vi "9205 Read 2.vi"(8 "error in":errorcluster, 11 "Module Config Selector":i16) -> (0 "error out":errorcluster, 3 "Data Array":sgl[](array[numeric]))   [LabVIEW 2015]
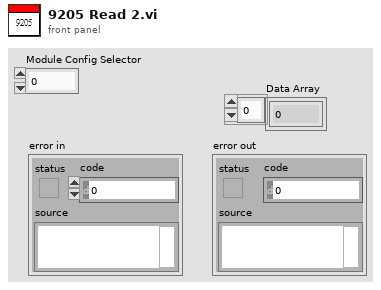
[diagram p1: front panel]
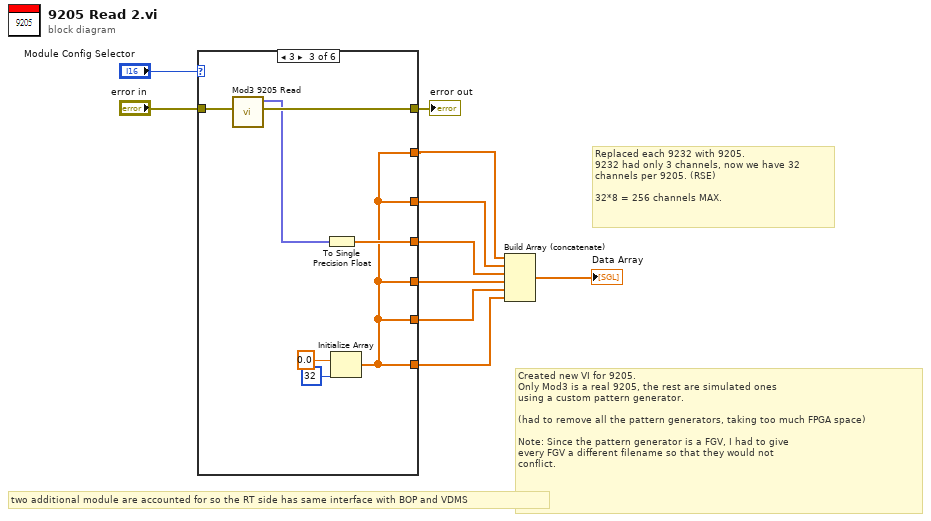
[diagram p0: block diagram]
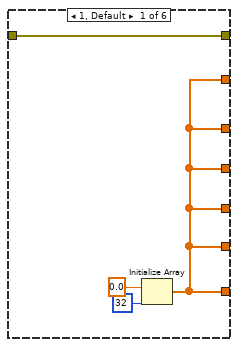
[diagram p2: hidden frame]
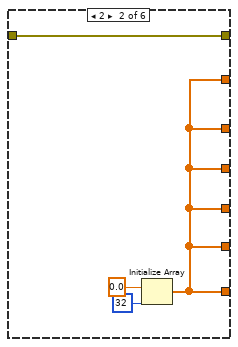
[diagram p3: hidden frame]
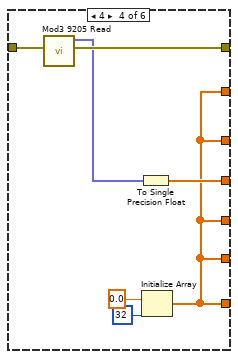
[diagram p4: hidden frame]
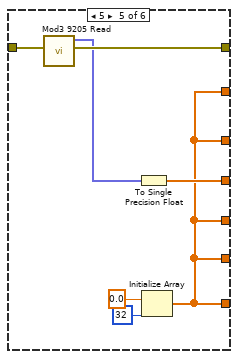
[diagram p5: hidden frame]
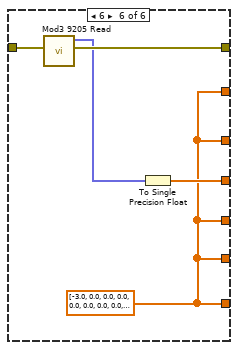
[diagram p6: hidden frame]
diagram:
  # "Replaced each 9232 with 9205.\n9232 had only 3 channels, now we have 32\nchannels per 9205. (RSE)\n\n32*8 = 256 channels MAX."
  # "Created new VI for 9205.\nOnly Mod3 is a real 9205, the rest are simulated ones\nusing a custom pattern generator.\n\n(had to remove all the pattern generators, taking too much FPGA space)\n\nNote: Since the pattern generator is a FGV, I had to give\nevery FGV a different filename so that they would not\nconflict."
  # "two additional module are accounted for so the RT side has same interface with BOP and VDMS"
  n1 = case shown="3" "Module Config Selector" {
    tunnel: "error in" -> [w12 w16 w25 w32 w39 w44]
    tunnel: [w12 w16 w24 w31 w38 w43] -> w9
    tunnel: [w11 w15 w20 w27 w34 w41] -> w6
    tunnel: [w11 w15 w19 w26 w33 w40] -> w5
    tunnel: [w11 w15 w19 w26 w33 w40] -> w4
    tunnel: [w11 w15 w19 w26 w33 w40] -> w3
    tunnel: [w11 w15 w19 w26 w33 w40] -> w2
    tunnel: [w11 w15 w19 w26 w33 w40] -> w1
    frame 1, Default {
      n2 = Initialize Array(sgl 0.0 ("element"), 32 ("dimension size")) -> (w11:sgl[])
    }
    frame 2 {
      n3 = Initialize Array(sgl 0.0 ("element"), 32 ("dimension size")) -> (w15:sgl[])
    }
    frame 3 {
      n4 = call "Mod3 9205 Read.vi"("error in"=w25) -> ("error out"=w24:errorcluster, "data out"=w21:fxp<+/-,26,5>[])  [unwired: 9 in]
      n5 = To Single Precision Float(number=w21) -> (single precision float=w20:sgl[])
      n6 = Initialize Array(sgl 0.0 ("element"), 32 ("dimension size")) -> (w19:sgl[])
    }
    frame 4 {
      n7 = call "Mod3 9205 Read.vi"("error in"=w32) -> ("error out"=w31:errorcluster, "data out"=w30:fxp<+/-,26,5>[])  [unwired: 9 in]
      n8 = To Single Precision Float(number=w30) -> (single precision float=w27:sgl[])
      n9 = Initialize Array(sgl 0.0 ("element"), 32 ("dimension size")) -> (w26:sgl[])
    }
    frame 5 {
      n10 = call "Mod3 9205 Read.vi"("error in"=w39) -> ("error out"=w38:errorcluster, "data out"=w37:fxp<+/-,26,5>[])  [unwired: 9 in]
      n11 = To Single Precision Float(number=w37) -> (single precision float=w34:sgl[])
      n12 = Initialize Array(sgl 0.0 ("element"), 32 ("dimension size")) -> (w33:sgl[])
    }
    frame 6 {
      w40 = sgl[] [-3.0, 0.0, 0.0, 0.0, 0.0, 0.0, 0.0, 0.0, 0.0, 0.0, 0.0, 0.0, 0.0, 0.0, 0.0, 0.0, 0.0, 0.0, 0.0, 0.0, 0.0, 0.0, 0.0, 0.0, 0.0, 0.0, 0.0, 0.0, 0.0, 0.0, 0.0, 0.0] ("Array")
      n13 = call "Mod3 9205 Read.vi"("error in"=w44) -> ("error out"=w43:errorcluster, "data out"=w42:fxp<+/-,26,5>[])  [unwired: 9 in]
      n14 = To Single Precision Float(number=w42) -> (single precision float=w41:sgl[])
    }
  }
  "error out" <- w9
  n15 = Build Array (concatenate)(w5, w4, w6, w3, w2, w1) -> (→"Data Array":sgl[])
